vi "Add_Shortcut.vi"(8 "error in (no error)":errorcluster, 9 "shortcutAddresses":T1[](array[typedef]), 10 "shortcut":refnum<class "IB_Shortcut.lvclass">, 11 "IB_Source_File in":refnum<class "IB_Source_File.lvclass">) -> (0 "error out":errorcluster, 1 "name change?":bool, 2 "shortcut":refnum<class "IB_Shortcut.lvclass">, 3 "IB_Source_File out":refnum<class "IB_Source_File.lvclass">)   [LabVIEW 2020, in "IB_Source_File.lvclass"]
uses:
  <vilib>/AppBuilder/IB_Classes/Source/File/IB_Source_File.lvclass
  <vilib>/AppBuilder/IB_Classes/Source/File/IB_Source_File.lvclass/IB_Source_File.ctl
  <vilib>/AppBuilder/IB_Classes/Shortcut/IB_Shortcut.lvclass
  <resource>/Framework/Providers/Builds/Installer/CDK_sTypeDef_ShortcutAddress.ctl
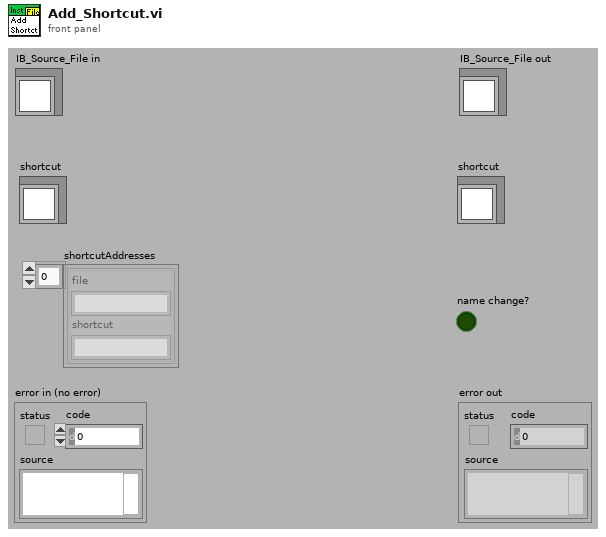
[diagram p1: front panel]
types:
  T1 = typedef "CDK_sTypeDef_ShortcutAddress.ctl" = cluster{"file":string, "shortcut":string}
  T2 = typedef "IB_Shortcut.ctl" = cluster{"name":string, "destIndex":i32, "subDir":string, "address":string}
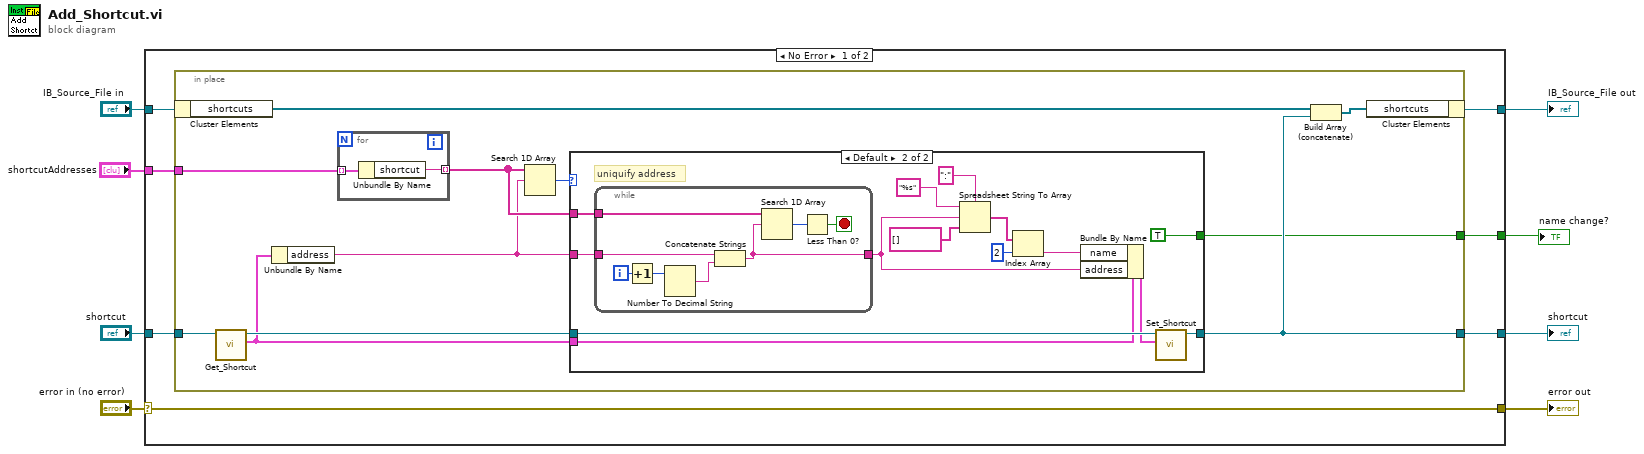
[diagram p0: block diagram]
diagram:
  n1 = case shown="No Error" "error in (no error)" {
    selector: "error in (no error)" -> [w15 w54]
    tunnel: [w15 w54] -> w7
    tunnel: "IB_Source_File in" -> [w14 w53]
    tunnel: "shortcut" -> [w12 w52]
    tunnel: [w13 w53] -> w4
    tunnel: [w11 w52] -> w3
    tunnel: [w10 _] -> w2
    tunnel: "shortcutAddresses" -> [w9 _]
    frame No Error {
      n2 = in-place {
        in-place-border: w12 -> [w24]
        in-place-border: [w19] -> w11
        in-place-border: [w18] -> w10
        in-place-border: w9 -> [w16]
        n3 = in-place-cluster #1(w14) -> ("shortcuts"=w26:refnum<class "IB_Shortcut.lvclass">[])
        n4 = call <vilib>:"Get_Shortcut.vi"("Class in"=w24) -> ("data"=w20:T2, "Class out"=w21:refnum<class "IB_Shortcut.lvclass">)  [unwired: 1 in, 8 out]
        n5 = Unbundle By Name(w20) -> ("address"=w17:string)
        n6 = for {
          tunnel: w16 -> [w50] mode=indexing
          tunnel: [w51] -> w23 mode=indexing
          n7 = Unbundle By Name(w50) -> ("shortcut"=w51:string)
        }
        n8 = Search 1D Array(1D array=w23, element=w17) -> (index of element=w22:i32)  [unwired: 1 out]
        n9 = case shown="Default" w22 {
          tunnel: w23 -> [_ w41]
          tunnel: w17 -> [_ w40]
          tunnel: w21 -> [w27 w39]
          tunnel: w20 -> [_ w38]
          tunnel: [w27 w36] -> w19
          tunnel: [_ TRUE] -> w18
          frame -1 {
          }
          frame Default {
            # "uniquify address"
            n10 = while {
              tunnel: w40 -> [w46]
              tunnel: w41 -> [w45]
              tunnel: [w42] -> w29
              i -> [w49]
              stop <- w43 stop-if-true
              n11 = Increment(x=w49) -> (x+1=w48:i32)
              n12 = Number To Decimal String(number=w48) -> (decimal integer string=w47:string)  [unwired: 1 out]
              n13 = Concatenate Strings(w46, w47) -> (w42:string)
              n14 = Search 1D Array(1D array=w45, element=w42) -> (index of element=w44:i32)  [unwired: 1 out]
              n15 = Less Than 0?(x=w44) -> (x < 0?=w43:bool)
            }
            n16 = Spreadsheet String To Array(delimiter (Tab)=":", format string="%s", spreadsheet string=w29, array type (2D Dbl)=string[] []) -> (array=w33:string[])
            n17 = Index Array(array=w33, index=2) -> (element=w28:string)
            n18 = Bundle By Name(cluster=w38, "name"=w28, "address"=w29) -> (w37:T2)
            n19 = call <vilib>:"Set_Shortcut.vi"("data"=w37, "Class in"=w39) -> ("Class out"=w36:refnum<class "IB_Shortcut.lvclass">)  [unwired: 1 in, 8 out]
          }
        }
        n20 = Build Array (concatenate)(w26, w19) -> (w25:refnum<class "IB_Shortcut.lvclass">[])
        n21 = in-place-cluster #1("shortcuts"=w25) -> (w13:refnum<class "IB_Source_File.lvclass">)
      }
    }
    frame Error {
    }
  }
  "error out" <- w7
  "IB_Source_File out" <- w4
  "shortcut" <- w3
  "name change?" <- w2
